vi "Get ID.vi"(11 "Challenge in":refnum<class "Challenge.lvclass">) -> (2 "ID":i64, 3 "Challenge out":refnum<class "Challenge.lvclass">)   [LabVIEW 2020, in "Summer of LabVIEW.lvlib" / "Challenge.lvclass"]
uses:
  Challenge.lvclass
  Challenge.lvclass/Challenge.ctl
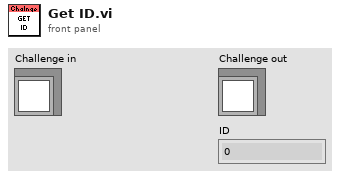
[diagram p1: front panel]
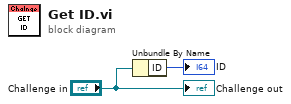
[diagram p0: block diagram]
diagram:
  n1 = Unbundle By Name("Challenge in") -> ("ID"=→"ID":i64)
  "Challenge out" <- "Challenge in"
